vi "visualise sand.vi"(11 "Array in":cluster{"x":i32, "y":i32}[](array[cluster])) -> (3 "Array out":bool[][](array[boolean]))   [LabVIEW 2019]
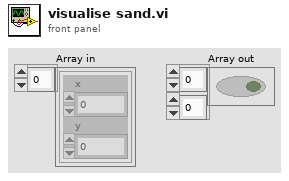
[diagram p1: front panel]
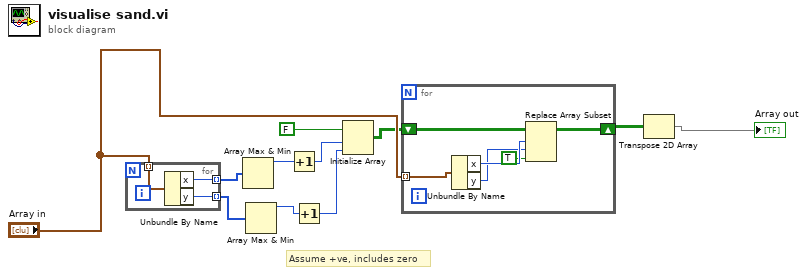
[diagram p0: block diagram]
diagram:
  # "Assume +ve, includes zero"
  n1 = for {
    tunnel: "Array in" -> [w14] mode=indexing
    tunnel: [w13] -> w6 mode=indexing
    tunnel: [w12] -> w7 mode=indexing
    n2 = Unbundle By Name(w14) -> ("x"=w13:i32, "y"=w12:i32)
  }
  n3 = Array Max & Min(array=w6) -> (max value=w4:i32)  [unwired: 3 out]
  n4 = Array Max & Min(array=w7) -> (max value=w2:i32)  [unwired: 3 out]
  n5 = Increment(x=w4) -> (x+1=w3:i32)
  n6 = Increment(x=w2) -> (x+1=w1:i32)
  n7 = Initialize Array(FALSE, w3, w1) -> (w8:bool[][])
  n8 = for {
    tunnel: "Array in" -> [w19] mode=indexing
    shift-right: [w15] -> w10
    shift-left: w8 -> [w20]
    n9 = Unbundle By Name(w19) -> ("x"=w18:i32, "y"=w17:i32)
    n10 = Replace Array Subset(array=w20, new element=TRUE ("new element/subarray"), index (row)=w18, index (col)=w17) -> (w15:bool[][])
  }
  n11 = Transpose 2D Array(2D array=w10) -> (transposed array=→"Array out":bool[][])
